vi "Bar Code Reader_v3.vi"() -> ()   [LabVIEW 2016]
uses:
  <vilib>/NXT/Block Support/NXT_OutputPort.ctl
  <vilib>/NXT/Block Support/NXT_InputPort.ctl
  <vilib>/NXT/Dual Mode Library/Sensors/EV3_Color_Color.vi
  <vilib>/NXT/NXTIO Xnodes/NXTIONodeSubVIs/NXTMoveMotors.vi
  <vilib>/NXT/NXTIO Xnodes/NXTIONodeSubVIs/NXTMotorRunDistance.vi
  <vilib>/NXT/Dual Mode Library/Waits/Wait_Num.vi
  <vilib>/NXT/Subs/LVHSConnector.ctl
  <vilib>/NXT/NXTIO Xnodes/AddressXNode/NXTIOAddress.xnode
  <vilib>/NXT/NXTIO Xnodes/NXTIOXNode/NXTIO.xnode
  <vilib>/NXT/LegoClasses/BrickReference/BrickReference.lvclass
panel:
  out "Error Message":string
  out "Total Marbles":dbl
  out "Small/HDPE 4":dbl
  out "Large/Steel 4":dbl
  out "Material 4":string
  out "Small/HDPE 3":dbl
  out "Large/Steel 3":dbl
  out "Material 3":string
  out "Small/HDPE 2":dbl
  out "Large/Steel 2":dbl
  out "Material 2":string
  out "Small/HDPE 1":dbl
  out "Large/Steel 1":dbl
  out "String 3":string
  out "String 2":string
  out "Material 1":string
  out "String":string
  out "Numeric":dbl
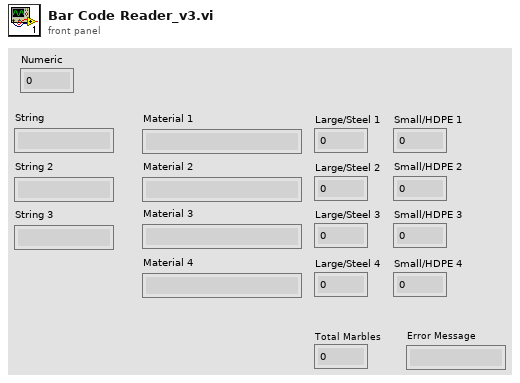
[diagram p1: front panel]
types:
  T1 = typedef "ColorSensorColors.ctl" = enum16{"No Color", "Black", "Blue", "Green", "Yellow", "Red", "White", "Brown"}
  T2 = typedef "NXT_OutputPort.ctl" = u8
  T3 = typedef "LVHSConnector.ctl" = refnum<class "BrickReference.lvclass">
  T4 = typedef "NXT_InputPort.ctl" = u32
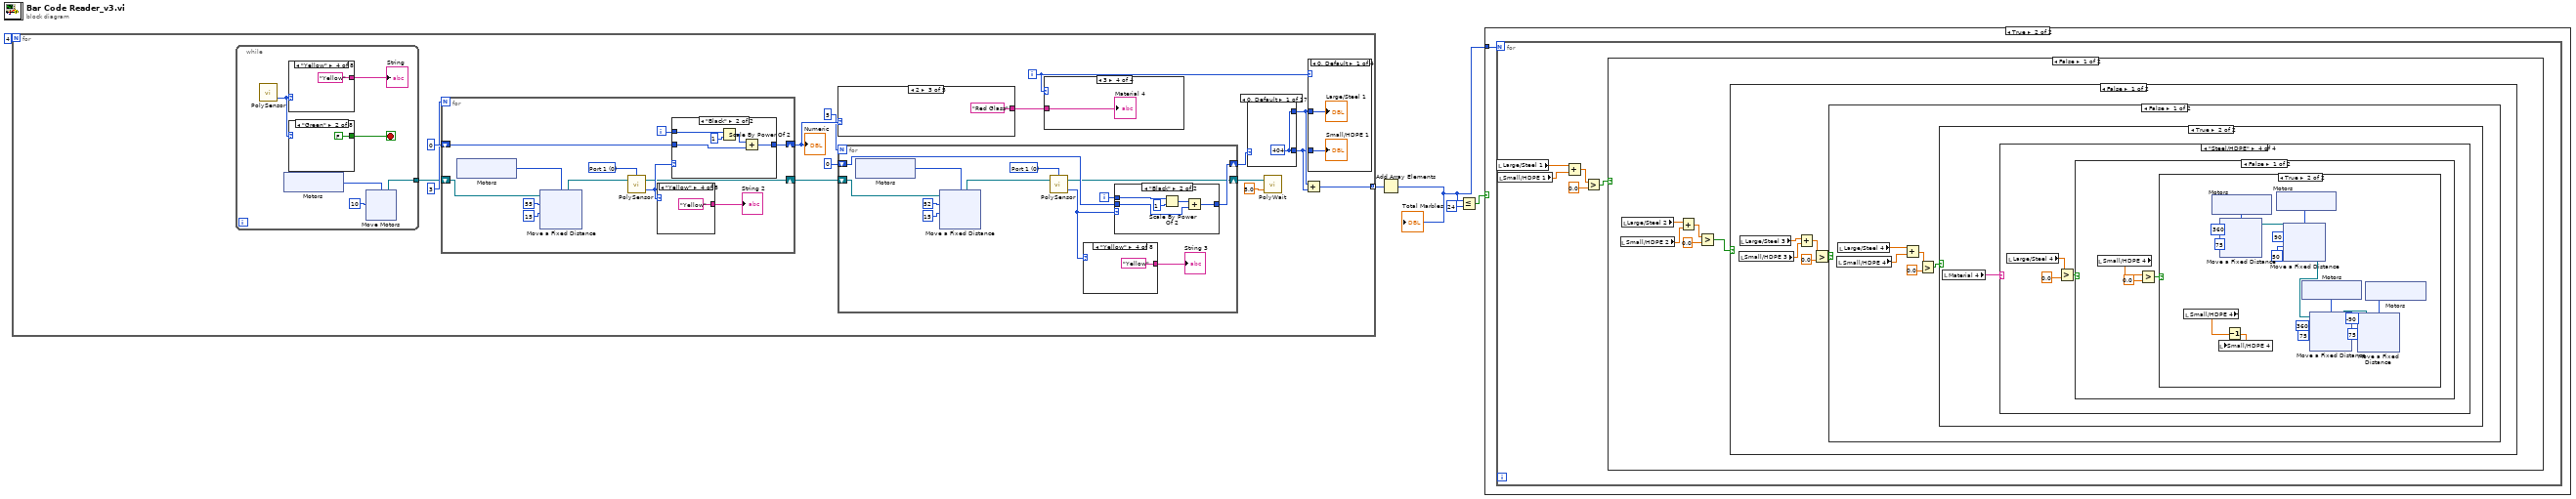
[diagram p0: block diagram]
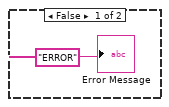
[diagram p2: hidden frame]
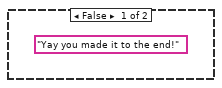
[diagram p3: hidden frame]
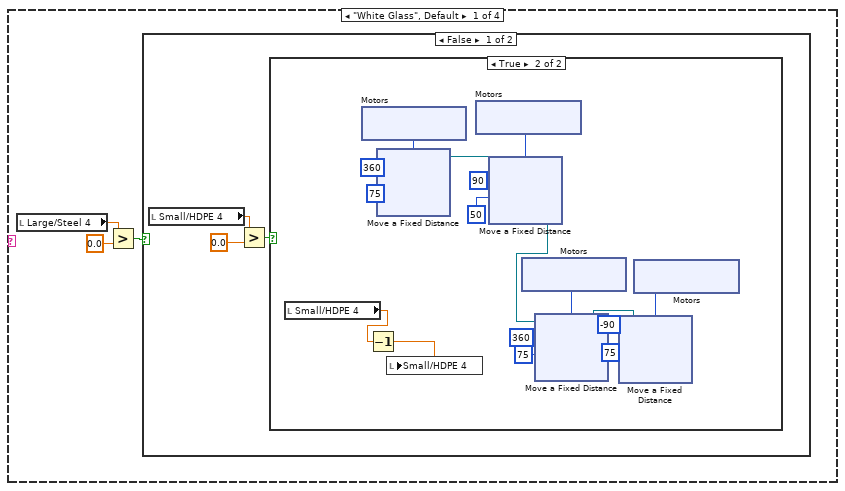
[diagram p4: hidden frame]
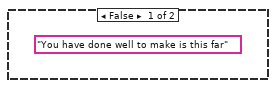
[diagram p5: hidden frame]
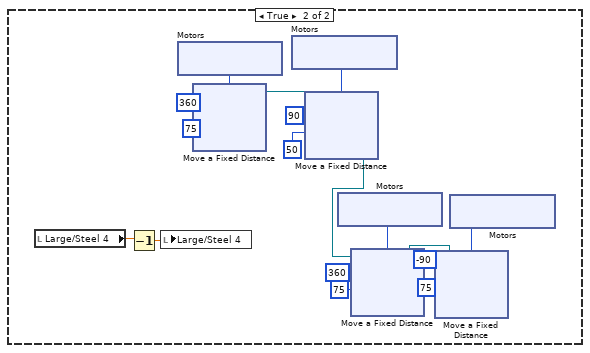
[diagram p6: hidden frame]
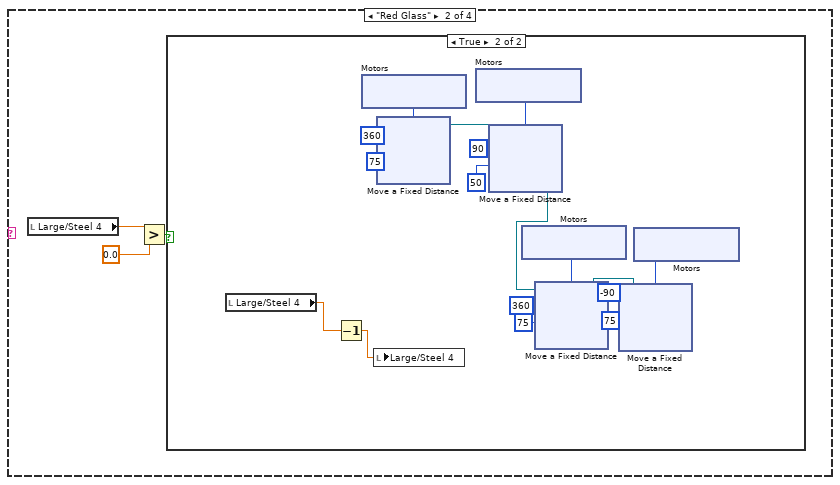
[diagram p7: hidden frame]
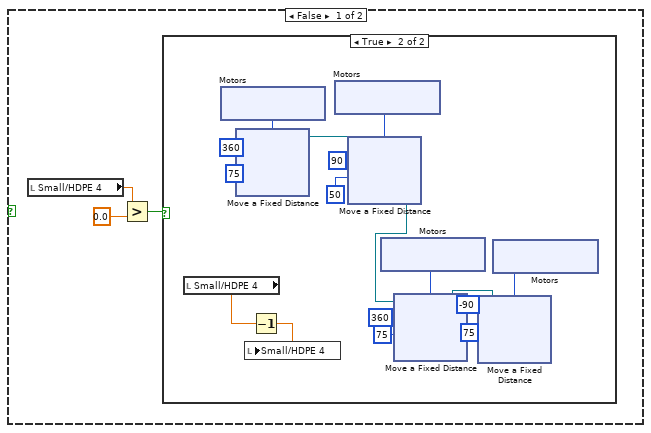
[diagram p8: hidden frame]
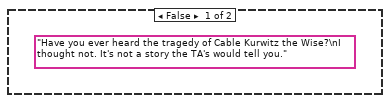
[diagram p9: hidden frame]
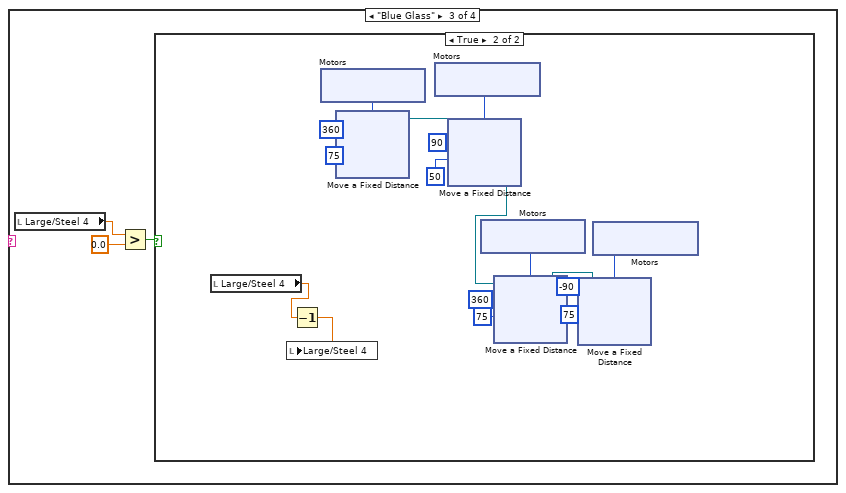
[diagram p10: hidden frame]
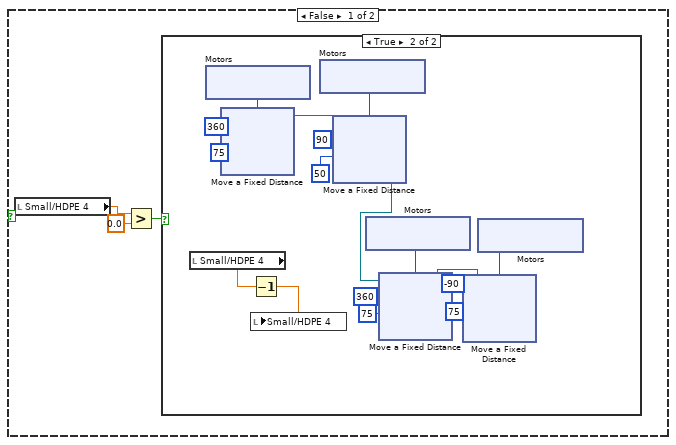
[diagram p11: hidden frame]
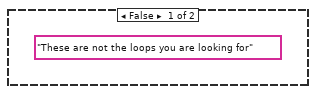
[diagram p12: hidden frame]
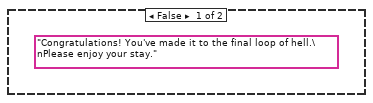
[diagram p13: hidden frame]
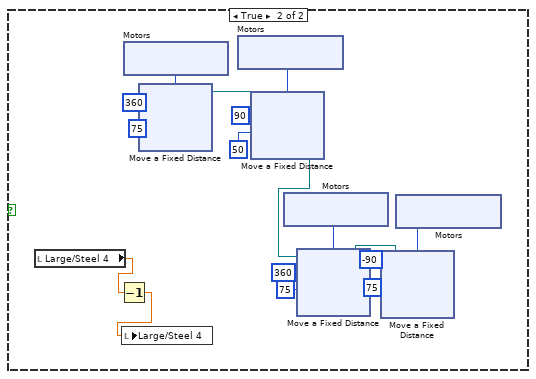
[diagram p14: hidden frame]
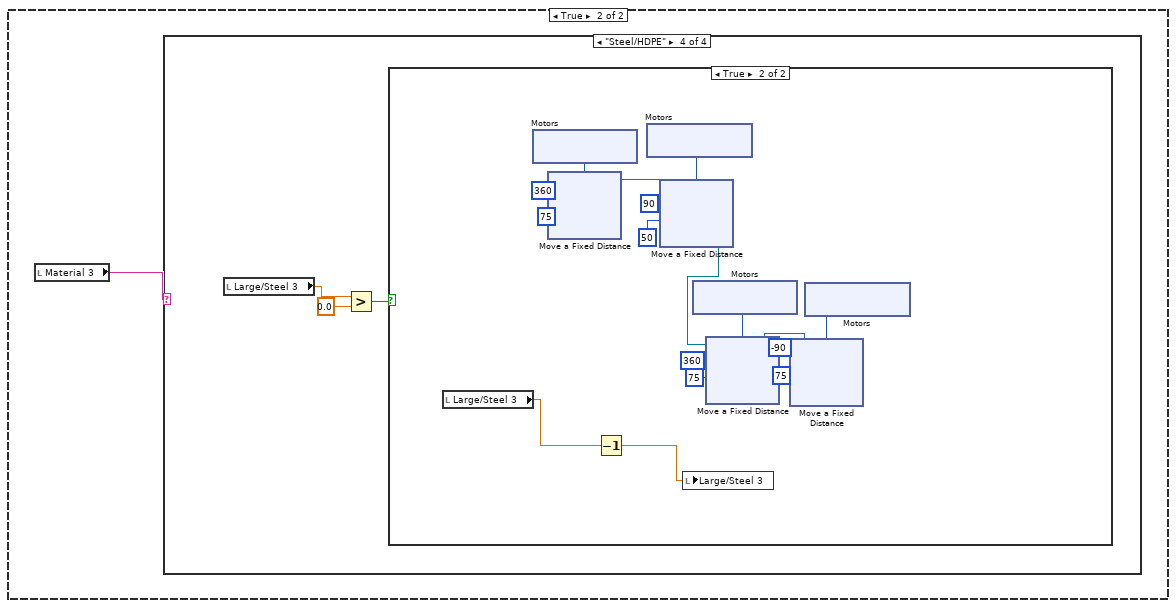
[diagram p15: hidden frame]
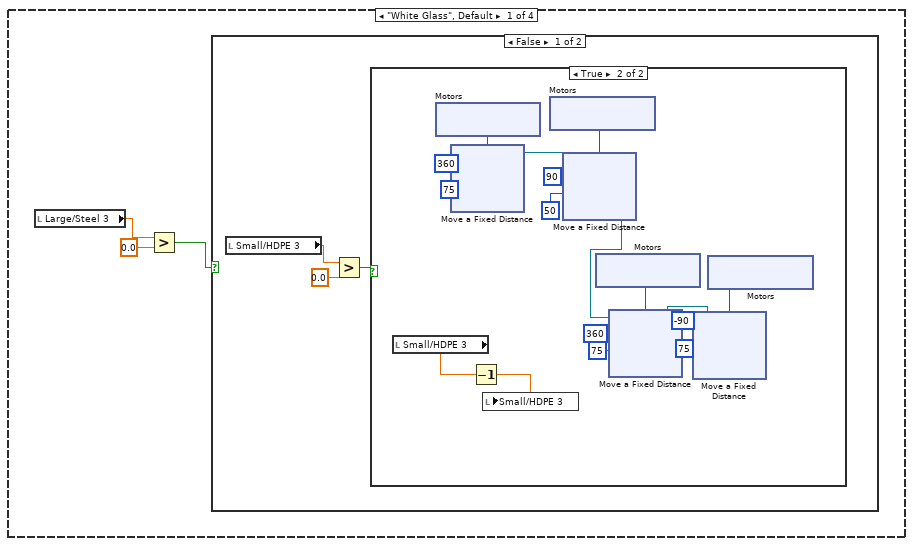
[diagram p16: hidden frame]
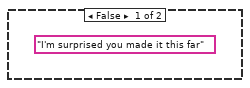
[diagram p17: hidden frame]
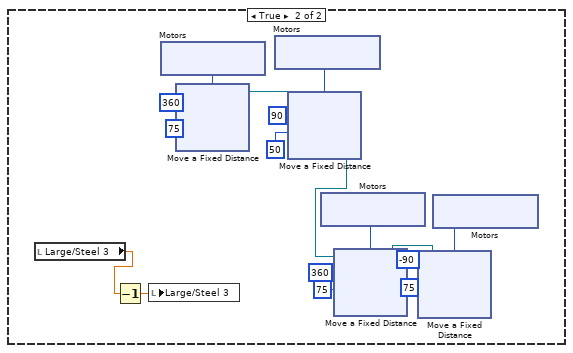
[diagram p18: hidden frame]
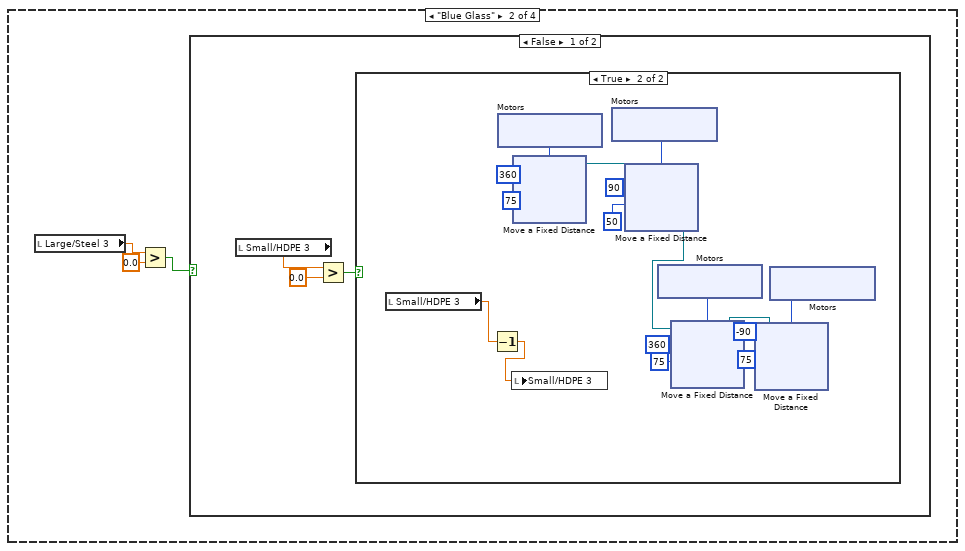
[diagram p19: hidden frame]
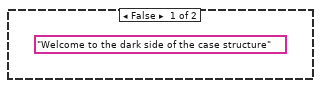
[diagram p20: hidden frame]
diagram:
  n1 = for {
    N: 4 -> [_]
    tunnel: [w6] -> w4 mode=indexing
    i -> [w11]
    n2 = while {
      tunnel: [w109] -> w18
      stop <- w113 stop-if-true
      n3 = call-poly <vilib>:"PolySensor.vi"() -> ("Detected Color"=w111:T1)  [unwired: 3 in, 1 out]
      n4 = xnode "Motors"() -> ("Motor"=w108:T2)
      n5 = case shown="\"Yellow\"" w111 {
        tunnel: ["No Color" "Blue" "Green" "Yellow" "Red" "White" "Brown" "Black"] -> w112
        frame "No Color", Default {
        }
        frame "Blue" {
        }
        frame "Green" {
        }
        frame "Yellow" {
        }
        frame "Red" {
        }
        frame "White" {
        }
        frame "Brown" {
        }
        frame "Black" {
        }
      }
      "String" <- w112
      n6 = case shown="\"Green\"" w111 {
        tunnel: [FALSE FALSE FALSE FALSE FALSE FALSE FALSE TRUE] -> w113
        frame "No Color", Default {
        }
        frame "Green" {
        }
        frame "Yellow" {
        }
        frame "Red" {
        }
        frame "White" {
        }
        frame "Brown" {
        }
        frame "Blue" {
        }
        frame "Black" {
        }
      }
      n7 = xnode "Move Motors"("Power/Speed 1"=i8 10, "Motors"=w108) -> ("NXT/EV3"=w109:T3)  [unwired: 1 in]
    }
    n8 = for {
      N: 3 -> [_]
      shift-right: [w149] -> w17
      shift-left: 0 -> [w148]
      shift-right: [w144] -> w13
      shift-left: w18 -> [w141]
      i -> [w145]
      w138 = T4 0 items=["Port 1", "Port 2", "Port 3", "Port 4"] ("Port (Port 1)")
      n9 = xnode "Motors"() -> ("Motor"=w139:T2)
      n10 = xnode "Move a Fixed Distance"("Speed 1"=i8 15, "Distance 1"=55, "Motors"=w139, "NXT/EV3"=w141) -> ("NXT/EV3"=w140:T3)
      n11 = call-poly <vilib>:"PolySensor.vi"("NXT/EV3"=w140, "Port (Port 1)"=w138) -> ("Detected Color"=w146:T1, "NXT/EV3"=w144:T3)  [unwired: 1 in]
      n12 = case shown="\"Yellow\"" w146 {
        tunnel: ["No Color" "Blue" "Green" "Yellow" "Red" "White" "Brown" "Black"] -> w147
        frame "No Color", Default {
        }
        frame "Blue" {
        }
        frame "Green" {
        }
        frame "Yellow" {
        }
        frame "Red" {
        }
        frame "White" {
        }
        frame "Brown" {
        }
        frame "Black" {
        }
      }
      "String 2" <- w147
      n13 = case shown="\"Black\"" w146 {
        tunnel: w145 -> [_ w173]
        tunnel: [w169 w171] -> w149
        tunnel: w148 -> [w169 w170]
        frame "White", Default {
        }
        frame "Black" {
          n14 = Scale By Power Of 2(n=w173, x=1) -> (x*2^n=w172:i32)
          n15 = Add(x=w172, y=w170) -> (x+y=w171:i32)
        }
      }
    }
    "Numeric" <- w17
    n16 = case shown="2" w17 {
      tunnel: ["Something has gone wrong" "White Glass" "Red Glass" "Blue Glass" "Steel/HDPE"] -> w16
      frame 0, Default {
      }
      frame 1 {
      }
      frame 2 {
      }
      frame 3 {
      }
      frame 4 {
      }
    }
    n17 = for {
      N: 5 -> [_]
      shift-right: [w77] -> w12
      shift-left: 0 -> [w76]
      shift-right: [w72] -> w10
      shift-left: w13 -> [w69]
      i -> [w73]
      w66 = T4 0 items=["Port 1", "Port 2", "Port 3", "Port 4"] ("Port (Port 1)")
      n18 = xnode "Motors"() -> ("Motor"=w67:T2)
      n19 = xnode "Move a Fixed Distance"("Speed 1"=i8 15, "Distance 1"=52, "Motors"=w67, "NXT/EV3"=w69) -> ("NXT/EV3"=w68:T3)
      n20 = call-poly <vilib>:"PolySensor.vi"("NXT/EV3"=w68, "Port (Port 1)"=w66) -> ("Detected Color"=w74:T1, "NXT/EV3"=w72:T3)  [unwired: 1 in]
      n21 = case shown="\"Yellow\"" w74 {
        tunnel: ["No Color" "Blue" "Green" "Yellow" "Red" "White" "Brown" "Black"] -> w75
        frame "No Color", Default {
        }
        frame "Blue" {
        }
        frame "Green" {
        }
        frame "Yellow" {
        }
        frame "Red" {
        }
        frame "White" {
        }
        frame "Brown" {
        }
        frame "Black" {
        }
      }
      "String 3" <- w75
      n22 = case shown="\"Black\"" w74 {
        tunnel: w73 -> [_ w101]
        tunnel: [w97 w99] -> w77
        tunnel: w76 -> [w97 w98]
        frame "White", Default {
        }
        frame "Black" {
          n23 = Scale By Power Of 2(n=w101, x=1) -> (x*2^n=w100:i32)
          n24 = Add(x=w100, y=w98) -> (x+y=w99:i32)
        }
      }
    }
    n25 = case shown="3" w11 {
      tunnel: w16 -> [w29 w30 w31 w32]
      frame 0, Default {
        "Material 1" <- w29
      }
      frame 1 {
        "Material 2" <- w30
      }
      frame 2 {
        "Material 3" <- w31
      }
      frame 3 {
        "Material 4" <- w32
      }
    }
    n26 = case shown="0, Default" w12 {
      tunnel: [w33 0 1 2 3 0 1 2 3 0 1 2 3 0 1 2 3] -> w8
      tunnel: [w33 0 0 0 0 1 1 1 1 2 2 2 2 3 3 3 3] -> w7
      frame 0, Default {
        w33 = 404
      }
      frame 1 {
      }
      frame 2 {
      }
      frame 3 {
      }
      frame 4 {
      }
      frame 5 {
      }
      frame 6 {
      }
      frame 7 {
      }
      frame 8 {
      }
      frame 9 {
      }
      frame 10 {
      }
      frame 11 {
      }
      frame 12 {
      }
      frame 13 {
      }
      frame 14 {
      }
      frame 15 {
      }
      frame 16 {
      }
    }
    n27 = call-poly <vilib>:"PolyWait.vi"("Time (1 sec)"=sgl 5.0, "NXT/EV3"=w10) -> ()  [unwired: 2 in, 1 out]
    n28 = Add(x=w8, y=w7) -> (x+y=w6:i32)
    n29 = case shown="0, Default" w11 {
      tunnel: w8 -> [w22 w23 w25 w27]
      tunnel: w7 -> [w21 w24 w26 w28]
      frame 0, Default {
        "Small/HDPE 1" <- w21
        "Large/Steel 1" <- w22
      }
      frame 1 {
        "Large/Steel 2" <- w23
        "Small/HDPE 2" <- w24
      }
      frame 2 {
        "Large/Steel 3" <- w25
        "Small/HDPE 3" <- w26
      }
      frame 3 {
        "Large/Steel 4" <- w27
        "Small/HDPE 4" <- w28
      }
    }
  }
  n30 = Add Array Elements(numeric array=w4) -> (sum=w3:i32)
  "Total Marbles" <- w3
  n31 = Less Or Equal?(x=w3, y=24) -> (x <= y?=w1:bool)
  n32 = case shown="True" w1 {
    tunnel: w3 -> [_ w176]
    frame False {
      "Error Message" <- "ERROR"
    }
    frame True {
      n33 = for {
        N: w176 -> [_]
        n34 = local read "Large/Steel 1"() -> (w181:dbl)
        n35 = local read "Small/HDPE 1"() -> (w180:dbl)
        n36 = Add(x=w181, y=w180) -> (x+y=w179:dbl)
        n37 = Greater?(x=w179, y=0.0) -> (0:w177:bool)
        n38 = case shown="False" w177 {
          frame False {
            n39 = local read "Small/HDPE 2"() -> (w184:dbl)
            n40 = local read "Large/Steel 2"() -> (w183:dbl)
            n41 = Add(x=w183, y=w184) -> (x+y=w186:dbl)
            n42 = Greater?(x=w186, y=0.0) -> (0:w182:bool)
            n43 = case shown="False" w182 {
              frame False {
                n44 = local read "Small/HDPE 3"() -> (w188:dbl)
                n45 = local read "Large/Steel 3"() -> (w189:dbl)
                n46 = Add(x=w189, y=w188) -> (x+y=w191:dbl)
                n47 = Greater?(x=w191, y=0.0) -> (0:w187:bool)
                n48 = case shown="False" w187 {
                  frame False {
                    n49 = local read "Small/HDPE 4"() -> (w193:dbl)
                    n50 = local read "Large/Steel 4"() -> (w194:dbl)
                    n51 = Add(x=w194, y=w193) -> (x+y=w196:dbl)
                    n52 = Greater?(x=w196, y=0.0) -> (0:w192:bool)
                    n53 = case shown="True" w192 {
                      frame False {
                        (unwired) "Yay you made it to the end!"
                      }
                      frame True {
                        n54 = local read "Material 4"() -> (w197:string)
                        n55 = case shown="\"Steel/HDPE\"" w197 {
                          frame "White Glass", Default {
                            n56 = local read "Large/Steel 4"() -> (w199:dbl)
                            n57 = Greater?(x=w199, y=0.0) -> (0:w200:bool)
                            n58 = case shown="False" w200 {
                              frame False {
                                n59 = local read "Small/HDPE 4"() -> (w202:dbl)
                                n60 = Greater?(x=w202, y=0.0) -> (0:w203:bool)
                                n61 = case shown="True" w203 {
                                frame False {
                                (unwired) "You have done well to make is this far"
                                }
                                frame True {
                                n62 = local read "Small/HDPE 4"() -> (w205:dbl)
                                n63 = xnode "Motors"() -> ("Motor"=w206:T2)
                                n64 = Decrement(x=w205) -> (x-1=w204:dbl)
                                n65 = xnode "Move a Fixed Distance"("Speed 1"=i8 75, "Distance 1"=360, "Motors"=w206) -> ("NXT/EV3"=w209:T3)  [unwired: 1 in]
                                n66 = local write "Small/HDPE 4"(w204) -> ()
                                n67 = xnode "Motors"() -> ("Motor"=w210:T2)
                                n68 = xnode "Move a Fixed Distance"("Speed 1"=i8 50, "Distance 1"=90, "Motors"=w210, "NXT/EV3"=w209) -> ("NXT/EV3"=w220:T3)
                                n69 = xnode "Motors"() -> ("Motor"=w216:T2)
                                n70 = xnode "Move a Fixed Distance"("Speed 1"=i8 75, "Distance 1"=360, "Motors"=w216, "NXT/EV3"=w220) -> ("NXT/EV3"=w219:T3)
                                n71 = xnode "Motors"() -> ("Motor"=w213:T2)
                                n72 = xnode "Move a Fixed Distance"("Speed 1"=i8 75, "Distance 1"=-90, "Motors"=w213, "NXT/EV3"=w219) -> ()  [unwired: 1 out]
                                }
                                }
                              }
                              frame True {
                                n73 = local read "Large/Steel 4"() -> (w266:dbl)
                                n74 = Decrement(x=w266) -> (x-1=w265:dbl)
                                n75 = local write "Large/Steel 4"(w265) -> ()
                                n76 = xnode "Motors"() -> ("Motor"=w267:T2)
                                n77 = xnode "Move a Fixed Distance"("Speed 1"=i8 75, "Distance 1"=360, "Motors"=w267) -> ("NXT/EV3"=w270:T3)  [unwired: 1 in]
                                n78 = xnode "Motors"() -> ("Motor"=w271:T2)
                                n79 = xnode "Move a Fixed Distance"("Speed 1"=i8 50, "Distance 1"=90, "Motors"=w271, "NXT/EV3"=w270) -> ("NXT/EV3"=w281:T3)
                                n80 = xnode "Motors"() -> ("Motor"=w277:T2)
                                n81 = xnode "Move a Fixed Distance"("Speed 1"=i8 75, "Distance 1"=360, "Motors"=w277, "NXT/EV3"=w281) -> ("NXT/EV3"=w280:T3)
                                n82 = xnode "Motors"() -> ("Motor"=w274:T2)
                                n83 = xnode "Move a Fixed Distance"("Speed 1"=i8 75, "Distance 1"=-90, "Motors"=w274, "NXT/EV3"=w280) -> ()  [unwired: 1 out]
                              }
                            }
                          }
                          frame "Red Glass" {
                            n84 = local read "Large/Steel 4"() -> (w327:dbl)
                            n85 = Greater?(x=w327, y=0.0) -> (0:w328:bool)
                            n86 = case shown="True" w328 {
                              frame False {
                                n87 = local read "Small/HDPE 4"() -> (w329:dbl)
                                n88 = Greater?(x=w329, y=0.0) -> (0:w331:bool)
                                n89 = case shown="True" w331 {
                                frame False {
                                (unwired) "Have you ever heard the tragedy of Cable Kurwitz the Wise?\nI thought not. It's not a story the TA's would tell you."
                                }
                                frame True {
                                n90 = local read "Small/HDPE 4"() -> (w333:dbl)
                                n91 = xnode "Motors"() -> ("Motor"=w348:T2)
                                n92 = xnode "Move a Fixed Distance"("Speed 1"=i8 75, "Distance 1"=360, "Motors"=w348) -> ("NXT/EV3"=w345:T3)  [unwired: 1 in]
                                n93 = Decrement(x=w333) -> (x-1=w332:dbl)
                                n94 = local write "Small/HDPE 4"(w332) -> ()
                                n95 = xnode "Motors"() -> ("Motor"=w344:T2)
                                n96 = xnode "Move a Fixed Distance"("Speed 1"=i8 50, "Distance 1"=90, "Motors"=w344, "NXT/EV3"=w345) -> ("NXT/EV3"=w334:T3)
                                n97 = xnode "Motors"() -> ("Motor"=w338:T2)
                                n98 = xnode "Move a Fixed Distance"("Speed 1"=i8 75, "Distance 1"=360, "Motors"=w338, "NXT/EV3"=w334) -> ("NXT/EV3"=w335:T3)
                                n99 = xnode "Motors"() -> ("Motor"=w341:T2)
                                n100 = xnode "Move a Fixed Distance"("Speed 1"=i8 75, "Distance 1"=-90, "Motors"=w341, "NXT/EV3"=w335) -> ()  [unwired: 1 out]
                                }
                                }
                              }
                              frame True {
                                n101 = local read "Large/Steel 4"() -> (w394:dbl)
                                n102 = Decrement(x=w394) -> (x-1=w393:dbl)
                                n103 = xnode "Motors"() -> ("Motor"=w395:T2)
                                n104 = local write "Large/Steel 4"(w393) -> ()
                                n105 = xnode "Move a Fixed Distance"("Speed 1"=i8 75, "Distance 1"=360, "Motors"=w395) -> ("NXT/EV3"=w398:T3)  [unwired: 1 in]
                                n106 = xnode "Motors"() -> ("Motor"=w399:T2)
                                n107 = xnode "Move a Fixed Distance"("Speed 1"=i8 50, "Distance 1"=90, "Motors"=w399, "NXT/EV3"=w398) -> ("NXT/EV3"=w409:T3)
                                n108 = xnode "Motors"() -> ("Motor"=w405:T2)
                                n109 = xnode "Move a Fixed Distance"("Speed 1"=i8 75, "Distance 1"=360, "Motors"=w405, "NXT/EV3"=w409) -> ("NXT/EV3"=w408:T3)
                                n110 = xnode "Motors"() -> ("Motor"=w402:T2)
                                n111 = xnode "Move a Fixed Distance"("Speed 1"=i8 75, "Distance 1"=-90, "Motors"=w402, "NXT/EV3"=w408) -> ()  [unwired: 1 out]
                              }
                            }
                          }
                          frame "Blue Glass" {
                            n112 = local read "Large/Steel 4"() -> (w456:dbl)
                            n113 = Greater?(x=w456, y=0.0) -> (0:w455:bool)
                            n114 = case shown="True" w455 {
                              frame False {
                                n115 = local read "Small/HDPE 4"() -> (w458:dbl)
                                n116 = Greater?(x=w458, y=0.0) -> (0:w459:bool)
                                n117 = case shown="True" w459 {
                                frame False {
                                (unwired) "These are not the loops you are looking for"
                                }
                                frame True {
                                n118 = local read "Small/HDPE 4"() -> (w461:dbl)
                                n119 = xnode "Motors"() -> ("Motor"=w462:T2)
                                n120 = xnode "Move a Fixed Distance"("Speed 1"=i8 75, "Distance 1"=360, "Motors"=w462) -> ("NXT/EV3"=w465:T3)  [unwired: 1 in]
                                n121 = Decrement(x=w461) -> (x-1=w460:dbl)
                                n122 = local write "Small/HDPE 4"(w460) -> ()
                                n123 = xnode "Motors"() -> ("Motor"=w466:T2)
                                n124 = xnode "Move a Fixed Distance"("Speed 1"=i8 50, "Distance 1"=90, "Motors"=w466, "NXT/EV3"=w465) -> ("NXT/EV3"=w476:T3)
                                n125 = xnode "Motors"() -> ("Motor"=w472:T2)
                                n126 = xnode "Move a Fixed Distance"("Speed 1"=i8 75, "Distance 1"=360, "Motors"=w472, "NXT/EV3"=w476) -> ("NXT/EV3"=w475:T3)
                                n127 = xnode "Motors"() -> ("Motor"=w469:T2)
                                n128 = xnode "Move a Fixed Distance"("Speed 1"=i8 75, "Distance 1"=-90, "Motors"=w469, "NXT/EV3"=w475) -> ()  [unwired: 1 out]
                                }
                                }
                              }
                              frame True {
                                n129 = local read "Large/Steel 4"() -> (w522:dbl)
                                n130 = Decrement(x=w522) -> (x-1=w521:dbl)
                                n131 = local write "Large/Steel 4"(w521) -> ()
                                n132 = xnode "Motors"() -> ("Motor"=w523:T2)
                                n133 = xnode "Move a Fixed Distance"("Speed 1"=i8 75, "Distance 1"=360, "Motors"=w523) -> ("NXT/EV3"=w526:T3)  [unwired: 1 in]
                                n134 = xnode "Motors"() -> ("Motor"=w527:T2)
                                n135 = xnode "Move a Fixed Distance"("Speed 1"=i8 50, "Distance 1"=90, "Motors"=w527, "NXT/EV3"=w526) -> ("NXT/EV3"=w537:T3)
                                n136 = xnode "Motors"() -> ("Motor"=w533:T2)
                                n137 = xnode "Move a Fixed Distance"("Speed 1"=i8 75, "Distance 1"=360, "Motors"=w533, "NXT/EV3"=w537) -> ("NXT/EV3"=w536:T3)
                                n138 = xnode "Motors"() -> ("Motor"=w530:T2)
                                n139 = xnode "Move a Fixed Distance"("Speed 1"=i8 75, "Distance 1"=-90, "Motors"=w530, "NXT/EV3"=w536) -> ()  [unwired: 1 out]
                              }
                            }
                          }
                          frame "Steel/HDPE" {
                            n140 = local read "Large/Steel 4"() -> (w583:dbl)
                            n141 = Greater?(x=w583, y=0.0) -> (0:w584:bool)
                            n142 = case shown="False" w584 {
                              frame False {
                                n143 = local read "Small/HDPE 4"() -> (w586:dbl)
                                n144 = Greater?(x=w586, y=0.0) -> (0:w587:bool)
                                n145 = case shown="True" w587 {
                                frame False {
                                (unwired) "Congratulations! You've made it to the final loop of hell.\nPlease enjoy your stay."
                                }
                                frame True {
                                n146 = local read "Small/HDPE 4"() -> (w589:dbl)
                                n147 = xnode "Motors"() -> ("Motor"=w590:T2)
                                n148 = xnode "Move a Fixed Distance"("Speed 1"=i8 75, "Distance 1"=360, "Motors"=w590) -> ("NXT/EV3"=w593:T3)  [unwired: 1 in]
                                n149 = Decrement(x=w589) -> (x-1=w588:dbl)
                                n150 = local write "Small/HDPE 4"(w588) -> ()
                                n151 = xnode "Motors"() -> ("Motor"=w594:T2)
                                n152 = xnode "Move a Fixed Distance"("Speed 1"=i8 50, "Distance 1"=90, "Motors"=w594, "NXT/EV3"=w593) -> ("NXT/EV3"=w604:T3)
                                n153 = xnode "Motors"() -> ("Motor"=w600:T2)
                                n154 = xnode "Move a Fixed Distance"("Speed 1"=i8 75, "Distance 1"=360, "Motors"=w600, "NXT/EV3"=w604) -> ("NXT/EV3"=w603:T3)
                                n155 = xnode "Motors"() -> ("Motor"=w597:T2)
                                n156 = xnode "Move a Fixed Distance"("Speed 1"=i8 75, "Distance 1"=-90, "Motors"=w597, "NXT/EV3"=w603) -> ()  [unwired: 1 out]
                                }
                                }
                              }
                              frame True {
                                n157 = local read "Large/Steel 4"() -> (w650:dbl)
                                n158 = Decrement(x=w650) -> (x-1=w649:dbl)
                                n159 = local write "Large/Steel 4"(w649) -> ()
                                n160 = xnode "Motors"() -> ("Motor"=w651:T2)
                                n161 = xnode "Move a Fixed Distance"("Speed 1"=i8 75, "Distance 1"=360, "Motors"=w651) -> ("NXT/EV3"=w654:T3)  [unwired: 1 in]
                                n162 = xnode "Motors"() -> ("Motor"=w655:T2)
                                n163 = xnode "Move a Fixed Distance"("Speed 1"=i8 50, "Distance 1"=90, "Motors"=w655, "NXT/EV3"=w654) -> ("NXT/EV3"=w665:T3)
                                n164 = xnode "Motors"() -> ("Motor"=w661:T2)
                                n165 = xnode "Move a Fixed Distance"("Speed 1"=i8 75, "Distance 1"=360, "Motors"=w661, "NXT/EV3"=w665) -> ("NXT/EV3"=w664:T3)
                                n166 = xnode "Motors"() -> ("Motor"=w658:T2)
                                n167 = xnode "Move a Fixed Distance"("Speed 1"=i8 75, "Distance 1"=-90, "Motors"=w658, "NXT/EV3"=w664) -> ()  [unwired: 1 out]
                              }
                            }
                          }
                        }
                      }
                    }
                  }
                  frame True {
                    n168 = local read "Material 3"() -> (w710:string)
                    n169 = case shown="\"Steel/HDPE\"" w710 {
                      frame "White Glass", Default {
                        n170 = local read "Large/Steel 3"() -> (w713:dbl)
                        n171 = Greater?(x=w713, y=0.0) -> (0:w711:bool)
                        n172 = case shown="False" w711 {
                          frame False {
                            n173 = local read "Small/HDPE 3"() -> (w715:dbl)
                            n174 = Greater?(x=w715, y=0.0) -> (0:w716:bool)
                            n175 = case shown="True" w716 {
                              frame False {
                                (unwired) "I'm surprised you made it this far"
                              }
                              frame True {
                                n176 = local read "Small/HDPE 3"() -> (w718:dbl)
                                n177 = xnode "Motors"() -> ("Motor"=w719:T2)
                                n178 = xnode "Move a Fixed Distance"("Speed 1"=i8 75, "Distance 1"=360, "Motors"=w719) -> ("NXT/EV3"=w722:T3)  [unwired: 1 in]
                                n179 = Decrement(x=w718) -> (x-1=w717:dbl)
                                n180 = local write "Small/HDPE 3"(w717) -> ()
                                n181 = xnode "Motors"() -> ("Motor"=w723:T2)
                                n182 = xnode "Move a Fixed Distance"("Speed 1"=i8 50, "Distance 1"=90, "Motors"=w723, "NXT/EV3"=w722) -> ("NXT/EV3"=w733:T3)
                                n183 = xnode "Motors"() -> ("Motor"=w729:T2)
                                n184 = xnode "Move a Fixed Distance"("Speed 1"=i8 75, "Distance 1"=360, "Motors"=w729, "NXT/EV3"=w733) -> ("NXT/EV3"=w732:T3)
                                n185 = xnode "Motors"() -> ("Motor"=w726:T2)
                                n186 = xnode "Move a Fixed Distance"("Speed 1"=i8 75, "Distance 1"=-90, "Motors"=w726, "NXT/EV3"=w732) -> ()  [unwired: 1 out]
                              }
                            }
                          }
                          frame True {
                            n187 = local read "Large/Steel 3"() -> (w779:dbl)
                            n188 = Decrement(x=w779) -> (x-1=w778:dbl)
                            n189 = local write "Large/Steel 3"(w778) -> ()
                            n190 = xnode "Motors"() -> ("Motor"=w780:T2)
                            n191 = xnode "Move a Fixed Distance"("Speed 1"=i8 75, "Distance 1"=360, "Motors"=w780) -> ("NXT/EV3"=w783:T3)  [unwired: 1 in]
                            n192 = xnode "Motors"() -> ("Motor"=w784:T2)
                            n193 = xnode "Move a Fixed Distance"("Speed 1"=i8 50, "Distance 1"=90, "Motors"=w784, "NXT/EV3"=w783) -> ("NXT/EV3"=w794:T3)
                            n194 = xnode "Motors"() -> ("Motor"=w790:T2)
                            n195 = xnode "Move a Fixed Distance"("Speed 1"=i8 75, "Distance 1"=360, "Motors"=w790, "NXT/EV3"=w794) -> ("NXT/EV3"=w793:T3)
                            n196 = xnode "Motors"() -> ("Motor"=w787:T2)
                            n197 = xnode "Move a Fixed Distance"("Speed 1"=i8 75, "Distance 1"=-90, "Motors"=w787, "NXT/EV3"=w793) -> ()  [unwired: 1 out]
                          }
                        }
                      }
                      frame "Blue Glass" {
                        n198 = local read "Large/Steel 3"() -> (w841:dbl)
                        n199 = Greater?(x=w841, y=0.0) -> (0:w839:bool)
                        n200 = case shown="False" w839 {
                          frame False {
                            n201 = local read "Small/HDPE 3"() -> (w844:dbl)
                            n202 = Greater?(x=w844, y=0.0) -> (0:w842:bool)
                            n203 = case shown="True" w842 {
                              frame False {
                                (unwired) "Welcome to the dark side of the case structure"
                              }
                              frame True {
                                n204 = local read "Small/HDPE 3"() -> (w846:dbl)
                                n205 = Decrement(x=w846) -> (x-1=w845:dbl)
                                n206 = xnode "Motors"() -> ("Motor"=w847:T2)
                                n207 = local write "Small/HDPE 3"(w845) -> ()
                                n208 = xnode "Move a Fixed Distance"("Speed 1"=i8 75, "Distance 1"=360, "Motors"=w847) -> ("NXT/EV3"=w850:T3)  [unwired: 1 in]
                                n209 = xnode "Motors"() -> ("Motor"=w851:T2)
                                n210 = xnode "Move a Fixed Distance"("Speed 1"=i8 50, "Distance 1"=90, "Motors"=w851, "NXT/EV3"=w850) -> ("NXT/EV3"=w861:T3)
                                n211 = xnode "Motors"() -> ("Motor"=w857:T2)
                                n212 = xnode "Move a Fixed Distance"("Speed 1"=i8 75, "Distance 1"=360, "Motors"=w857, "NXT/EV3"=w861) -> ("NXT/EV3"=w860:T3)
                                n213 = xnode "Motors"() -> ("Motor"=w854:T2)
                                n214 = xnode "Move a Fixed Distance"("Speed 1"=i8 75, "Distance 1"=-90, "Motors"=w854, "NXT/EV3"=w860) -> ()  [unwired: 1 out]
                              }
                            }
                          }
                          frame True {
                            n215 = local read "Large/Steel 3"() -> (w907:dbl)
                            n216 = xnode "Motors"() -> ("Motor"=w908:T2)
                            n217 = xnode "Move a Fixed Distance"("Speed 1"=i8 75, "Distance 1"=360, "Motors"=w908) -> ("NXT/EV3"=w911:T3)  [unwired: 1 in]
                            n218 = Decrement(x=w907) -> (x-1=w906:dbl)
                            n219 = local write "Large/Steel 3"(w906) -> ()
                            n220 = xnode "Motors"() -> ("Motor"=w912:T2)
                            n221 = xnode "Move a Fixed Distance"("Speed 1"=i8 50, "Distance 1"=90, "Motors"=w912, "NXT/EV3"=w911) -> ("NXT/EV3"=w922:T3)
                            n222 = xnode "Motors"() -> ("Motor"=w918:T2)
                            n223 = xnode "Move a Fixed Distance"("Speed 1"=i8 75, "Distance 1"=360, "Motors"=w918, "NXT/EV3"=w922) -> ("NXT/EV3"=w921:T3)
                            n224 = xnode "Motors"() -> ("Motor"=w915:T2)
                            n225 = xnode "Move a Fixed Distance"("Speed 1"=i8 75, "Distance 1"=-90, "Motors"=w915, "NXT/EV3"=w921) -> ()  [unwired: 1 out]
                          }
                        }
                      }
                      frame "Red Glass" {
                        n226 = local read "Large/Steel 3"() -> (w968:dbl)
                        n227 = Greater?(x=w968, y=0.0) -> (0:w969:bool)
                        n228 = case shown="True" w969 {
                          frame False {
                            n229 = local read "Small/HDPE 3"() -> (w971:dbl)
                            n230 = Greater?(x=w971, y=0.0) -> (0:w972:bool)
                            n231 = case shown="True" w972 {
                              frame False {
                                (unwired) "Two to the one to the one to the three"
                              }
                              frame True {
                                n232 = local read "Small/HDPE 3"() -> (w974:dbl)
                                n233 = Decrement(x=w974) -> (x-1=w973:dbl)
                                n234 = local write "Small/HDPE 3"(w973) -> ()
                                n235 = xnode "Motors"() -> ("Motor"=w975:T2)
                                n236 = xnode "Move a Fixed Distance"("Speed 1"=i8 75, "Distance 1"=360, "Motors"=w975) -> ("NXT/EV3"=w978:T3)  [unwired: 1 in]
                                n237 = xnode "Motors"() -> ("Motor"=w979:T2)
                                n238 = xnode "Move a Fixed Distance"("Speed 1"=i8 50, "Distance 1"=90, "Motors"=w979, "NXT/EV3"=w978) -> ("NXT/EV3"=w989:T3)
                                n239 = xnode "Motors"() -> ("Motor"=w985:T2)
                                n240 = xnode "Move a Fixed Distance"("Speed 1"=i8 75, "Distance 1"=360, "Motors"=w985, "NXT/EV3"=w989) -> ("NXT/EV3"=w988:T3)
                                n241 = xnode "Motors"() -> ("Motor"=w982:T2)
                                n242 = xnode "Move a Fixed Distance"("Speed 1"=i8 75, "Distance 1"=-90, "Motors"=w982, "NXT/EV3"=w988) -> ()  [unwired: 1 out]
                              }
                            }
                          }
                          frame True {
                            n243 = local read "Large/Steel 3"() -> (w1035:dbl)
                            n244 = Decrement(x=w1035) -> (x-1=w1034:dbl)
                            n245 = local write "Large/Steel 3"(w1034) -> ()
                            n246 = xnode "Motors"() -> ("Motor"=w1036:T2)
                            n247 = xnode "Move a Fixed Distance"("Speed 1"=i8 75, "Distance 1"=360, "Motors"=w1036) -> ("NXT/EV3"=w1039:T3)  [unwired: 1 in]
                            n248 = xnode "Motors"() -> ("Motor"=w1040:T2)
                            n249 = xnode "Move a Fixed Distance"("Speed 1"=i8 50, "Distance 1"=90, "Motors"=w1040, "NXT/EV3"=w1039) -> ("NXT/EV3"=w1050:T3)
                            n250 = xnode "Motors"() -> ("Motor"=w1046:T2)
                            n251 = xnode "Move a Fixed Distance"("Speed 1"=i8 75, "Distance 1"=360, "Motors"=w1046, "NXT/EV3"=w1050) -> ("NXT/EV3"=w1049:T3)
                            n252 = xnode "Motors"() -> ("Motor"=w1043:T2)
                            n253 = xnode "Move a Fixed Distance"("Speed 1"=i8 75, "Distance 1"=-90, "Motors"=w1043, "NXT/EV3"=w1049) -> ()  [unwired: 1 out]
                          }
                        }
                      }
                      frame "Steel/HDPE" {
                        n254 = local read "Large/Steel 3"() -> (w1096:dbl)
                        n255 = Greater?(x=w1096, y=0.0) -> (0:w1097:bool)
                        n256 = case shown="True" w1097 {
                          frame False {
                            n257 = local read "Small/HDPE 3"() -> (w1099:dbl)
                            n258 = Greater?(x=w1099, y=0.0) -> (0:w1100:bool)
                            n259 = case shown="True" w1100 {
                              frame False {
                                (unwired) "labview wouldnt let me copy the variables successfully\nso I had to write every single case structure by hand."
                              }
                              frame True {
                                n260 = local read "Small/HDPE 3"() -> (w1102:dbl)
                                n261 = xnode "Motors"() -> ("Motor"=w1117:T2)
                                n262 = Decrement(x=w1102) -> (x-1=w1101:dbl)
                                n263 = xnode "Move a Fixed Distance"("Speed 1"=i8 75, "Distance 1"=360, "Motors"=w1117) -> ("NXT/EV3"=w1114:T3)  [unwired: 1 in]
                                n264 = local write "Small/HDPE 3"(w1101) -> ()
                                n265 = xnode "Motors"() -> ("Motor"=w1113:T2)
                                n266 = xnode "Move a Fixed Distance"("Speed 1"=i8 50, "Distance 1"=90, "Motors"=w1113, "NXT/EV3"=w1114) -> ("NXT/EV3"=w1103:T3)
                                n267 = xnode "Motors"() -> ("Motor"=w1107:T2)
                                n268 = xnode "Move a Fixed Distance"("Speed 1"=i8 75, "Distance 1"=360, "Motors"=w1107, "NXT/EV3"=w1103) -> ("NXT/EV3"=w1104:T3)
                                n269 = xnode "Motors"() -> ("Motor"=w1110:T2)
                                n270 = xnode "Move a Fixed Distance"("Speed 1"=i8 75, "Distance 1"=-90, "Motors"=w1110, "NXT/EV3"=w1104) -> ()  [unwired: 1 out]
                              }
                            }
                          }
                          frame True {
                            n271 = local read "Large/Steel 3"() -> (w1163:dbl)
                            n272 = xnode "Motors"() -> ("Motor"=w1164:T2)
                            n273 = xnode "Move a Fixed Distance"("Speed 1"=i8 75, "Distance 1"=360, "Motors"=w1164) -> ("NXT/EV3"=w1167:T3)  [unwired: 1 in]
                            n274 = Decrement(x=w1163) -> (x-1=w1162:dbl)
                            n275 = xnode "Motors"() -> ("Motor"=w1168:T2)
                            n276 = xnode "Move a Fixed Distance"("Speed 1"=i8 50, "Distance 1"=90, "Motors"=w1168, "NXT/EV3"=w1167) -> ("NXT/EV3"=w1178:T3)
                            n277 = local write "Large/Steel 3"(w1162) -> ()
                            n278 = xnode "Motors"() -> ("Motor"=w1174:T2)
                            n279 = xnode "Move a Fixed Distance"("Speed 1"=i8 75, "Distance 1"=360, "Motors"=w1174, "NXT/EV3"=w1178) -> ("NXT/EV3"=w1177:T3)
                            n280 = xnode "Motors"() -> ("Motor"=w1171:T2)
                            n281 = xnode "Move a Fixed Distance"("Speed 1"=i8 75, "Distance 1"=-90, "Motors"=w1171, "NXT/EV3"=w1177) -> ()  [unwired: 1 out]
                          }
                        }
                      }
                    }
                  }
                }
              }
              frame True {
                n282 = local read "Material 2"() -> (w1223:string)
                n283 = case shown="\"Steel/HDPE\"" w1223 {
                  frame "White Glass", Default {
                    n284 = local read "Large/Steel 2"() -> (w1226:dbl)
                    n285 = Greater?(x=w1226, y=0.0) -> (0:w1224:bool)
                    n286 = case shown="True" w1224 {
                      frame False {
                        n287 = local read "Small/HDPE 2"() -> (w1229:dbl)
                        n288 = Greater?(x=w1229, y=0.0) -> (0:w1227:bool)
                        n289 = case shown="True" w1227 {
                          frame False {
                            (unwired) "howdy random TA"
                          }
                          frame True {
                            n290 = local read "Small/HDPE 2"() -> (w1231:dbl)
                            n291 = Decrement(x=w1231) -> (x-1=w1230:dbl)
                            n292 = xnode "Motors"() -> ("Motor"=w1246:T2)
                            n293 = xnode "Move a Fixed Distance"("Speed 1"=i8 75, "Distance 1"=360, "Motors"=w1246) -> ("NXT/EV3"=w1243:T3)  [unwired: 1 in]
                            n294 = local write "Small/HDPE 2"(w1230) -> ()
                            n295 = xnode "Motors"() -> ("Motor"=w1242:T2)
                            n296 = xnode "Move a Fixed Distance"("Speed 1"=i8 50, "Distance 1"=90, "Motors"=w1242, "NXT/EV3"=w1243) -> ("NXT/EV3"=w1232:T3)
                            n297 = xnode "Motors"() -> ("Motor"=w1236:T2)
                            n298 = xnode "Move a Fixed Distance"("Speed 1"=i8 75, "Distance 1"=360, "Motors"=w1236, "NXT/EV3"=w1232) -> ("NXT/EV3"=w1233:T3)
                            n299 = xnode "Motors"() -> ("Motor"=w1239:T2)
                            n300 = xnode "Move a Fixed Distance"("Speed 1"=i8 75, "Distance 1"=-90, "Motors"=w1239, "NXT/EV3"=w1233) -> ()  [unwired: 1 out]
                          }
                        }
                      }
                      frame True {
                        n301 = local read "Large/Steel 2"() -> (w1292:dbl)
                        n302 = Decrement(x=w1292) -> (x-1=w1291:dbl)
                        n303 = local write "Large/Steel 2"(w1291) -> ()
                        n304 = xnode "Motors"() -> ("Motor"=w1293:T2)
                        n305 = xnode "Move a Fixed Distance"("Speed 1"=i8 75, "Distance 1"=360, "Motors"=w1293) -> ("NXT/EV3"=w1296:T3)  [unwired: 1 in]
                        n306 = xnode "Motors"() -> ("Motor"=w1297:T2)
                        n307 = xnode "Move a Fixed Distance"("Speed 1"=i8 50, "Distance 1"=90, "Motors"=w1297, "NXT/EV3"=w1296) -> ("NXT/EV3"=w1307:T3)
                        n308 = xnode "Motors"() -> ("Motor"=w1303:T2)
                        n309 = xnode "Move a Fixed Distance"("Speed 1"=i8 75, "Distance 1"=360, "Motors"=w1303, "NXT/EV3"=w1307) -> ("NXT/EV3"=w1306:T3)
                        n310 = xnode "Motors"() -> ("Motor"=w1300:T2)
                        n311 = xnode "Move a Fixed Distance"("Speed 1"=i8 75, "Distance 1"=-90, "Motors"=w1300, "NXT/EV3"=w1306) -> ()  [unwired: 1 out]
                      }
                    }
                  }
                  frame "Blue Glass" {
                    n312 = local read "Large/Steel 2"() -> (w1354:dbl)
                    n313 = Greater?(x=w1354, y=0.0) -> (0:w1353:bool)
                    n314 = case shown="False" w1353 {
                      frame True {
                        n315 = local read "Large/Steel 2"() -> (w1356:dbl)
                        n316 = Decrement(x=w1356) -> (x-1=w1355:dbl)
                        n317 = local write "Large/Steel 2"(w1355) -> ()
                        n318 = xnode "Motors"() -> ("Motor"=w1357:T2)
                        n319 = xnode "Move a Fixed Distance"("Speed 1"=i8 75, "Distance 1"=360, "Motors"=w1357) -> ("NXT/EV3"=w1360:T3)  [unwired: 1 in]
                        n320 = xnode "Motors"() -> ("Motor"=w1361:T2)
                        n321 = xnode "Move a Fixed Distance"("Speed 1"=i8 50, "Distance 1"=90, "Motors"=w1361, "NXT/EV3"=w1360) -> ("NXT/EV3"=w1371:T3)
                        n322 = xnode "Motors"() -> ("Motor"=w1367:T2)
                        n323 = xnode "Move a Fixed Distance"("Speed 1"=i8 75, "Distance 1"=360, "Motors"=w1367, "NXT/EV3"=w1371) -> ("NXT/EV3"=w1370:T3)
                        n324 = xnode "Motors"() -> ("Motor"=w1364:T2)
                        n325 = xnode "Move a Fixed Distance"("Speed 1"=i8 75, "Distance 1"=-90, "Motors"=w1364, "NXT/EV3"=w1370) -> ()  [unwired: 1 out]
                      }
                      frame False {
                        n326 = local read "Small/HDPE 2"() -> (w1418:dbl)
                        n327 = Greater?(x=w1418, y=0.0) -> (0:w1416:bool)
                        n328 = case shown="False" w1416 {
                          frame False {
                            (unwired) "This statement is false"
                          }
                          frame True {
                            n329 = local read "Small/HDPE 2"() -> (w1420:dbl)
                            n330 = Decrement(x=w1420) -> (x-1=w1419:dbl)
                            n331 = xnode "Motors"() -> ("Motor"=w1421:T2)
                            n332 = local write "Small/HDPE 2"(w1419) -> ()
                            n333 = xnode "Move a Fixed Distance"("Speed 1"=i8 75, "Distance 1"=360, "Motors"=w1421) -> ("NXT/EV3"=w1424:T3)  [unwired: 1 in]
                            n334 = xnode "Motors"() -> ("Motor"=w1425:T2)
                            n335 = xnode "Move a Fixed Distance"("Speed 1"=i8 50, "Distance 1"=90, "Motors"=w1425, "NXT/EV3"=w1424) -> ("NXT/EV3"=w1435:T3)
                            n336 = xnode "Motors"() -> ("Motor"=w1431:T2)
                            n337 = xnode "Move a Fixed Distance"("Speed 1"=i8 75, "Distance 1"=360, "Motors"=w1431, "NXT/EV3"=w1435) -> ("NXT/EV3"=w1434:T3)
                            n338 = xnode "Motors"() -> ("Motor"=w1428:T2)
                            n339 = xnode "Move a Fixed Distance"("Speed 1"=i8 75, "Distance 1"=-90, "Motors"=w1428, "NXT/EV3"=w1434) -> ()  [unwired: 1 out]
                          }
                        }
                      }
                    }
                  }
                  frame "Red Glass" {
                    n340 = local read "Large/Steel 2"() -> (w1482:dbl)
                    n341 = Greater?(x=w1482, y=0.0) -> (0:w1480:bool)
                    n342 = case shown="False" w1480 {
                      frame False {
                        n343 = local read "Small/HDPE 2"() -> (w1485:dbl)
                        n344 = Greater?(x=w1485, y=0.0) -> (0:w1483:bool)
                        n345 = case shown="False" w1483 {
                          frame False {
                            (unwired) "I hate everything\n"
                          }
                          frame True {
                            n346 = local read "Small/HDPE 2"() -> (w1487:dbl)
                            n347 = xnode "Motors"() -> ("Motor"=w1488:T2)
                            n348 = xnode "Move a Fixed Distance"("Speed 1"=i8 75, "Distance 1"=360, "Motors"=w1488) -> ("NXT/EV3"=w1491:T3)  [unwired: 1 in]
                            n349 = Decrement(x=w1487) -> (x-1=w1486:dbl)
                            n350 = local write "Small/HDPE 2"(w1486) -> ()
                            n351 = xnode "Motors"() -> ("Motor"=w1492:T2)
                            n352 = xnode "Move a Fixed Distance"("Speed 1"=i8 50, "Distance 1"=90, "Motors"=w1492, "NXT/EV3"=w1491) -> ("NXT/EV3"=w1502:T3)
                            n353 = xnode "Motors"() -> ("Motor"=w1498:T2)
                            n354 = xnode "Move a Fixed Distance"("Speed 1"=i8 75, "Distance 1"=360, "Motors"=w1498, "NXT/EV3"=w1502) -> ("NXT/EV3"=w1501:T3)
                            n355 = xnode "Motors"() -> ("Motor"=w1495:T2)
                            n356 = xnode "Move a Fixed Distance"("Speed 1"=i8 75, "Distance 1"=-90, "Motors"=w1495, "NXT/EV3"=w1501) -> ()  [unwired: 1 out]
                          }
                        }
                      }
                      frame True {
                        n357 = local read "Large/Steel 2"() -> (w1548:dbl)
                        n358 = Decrement(x=w1548) -> (x-1=w1547:dbl)
                        n359 = local write "Large/Steel 2"(w1547) -> ()
                        n360 = xnode "Motors"() -> ("Motor"=w1549:T2)
                        n361 = xnode "Move a Fixed Distance"("Speed 1"=i8 75, "Distance 1"=360, "Motors"=w1549) -> ("NXT/EV3"=w1552:T3)  [unwired: 1 in]
                        n362 = xnode "Motors"() -> ("Motor"=w1553:T2)
                        n363 = xnode "Move a Fixed Distance"("Speed 1"=i8 50, "Distance 1"=90, "Motors"=w1553, "NXT/EV3"=w1552) -> ("NXT/EV3"=w1563:T3)
                        n364 = xnode "Motors"() -> ("Motor"=w1559:T2)
                        n365 = xnode "Move a Fixed Distance"("Speed 1"=i8 75, "Distance 1"=360, "Motors"=w1559, "NXT/EV3"=w1563) -> ("NXT/EV3"=w1562:T3)
                        n366 = xnode "Motors"() -> ("Motor"=w1556:T2)
                        n367 = xnode "Move a Fixed Distance"("Speed 1"=i8 75, "Distance 1"=-90, "Motors"=w1556, "NXT/EV3"=w1562) -> ()  [unwired: 1 out]
                      }
                    }
                  }
                  frame "Steel/HDPE" {
                    n368 = local read "Large/Steel 2"() -> (w1610:dbl)
                    n369 = Greater?(x=w1610, y=0.0) -> (0:w1608:bool)
                    n370 = case shown="False" w1608 {
                      frame False {
                        n371 = local read "Small/HDPE 2"() -> (w1613:dbl)
                        n372 = Greater?(x=w1613, y=0.0) -> (0:w1611:bool)
                        n373 = case shown="False" w1611 {
                          frame False {
                            (unwired) "I've lost all my marbles"
                          }
                          frame True {
                            n374 = local read "Small/HDPE 2"() -> (w1615:dbl)
                            n375 = xnode "Motors"() -> ("Motor"=w1616:T2)
                            n376 = xnode "Move a Fixed Distance"("Speed 1"=i8 75, "Distance 1"=360, "Motors"=w1616) -> ("NXT/EV3"=w1619:T3)  [unwired: 1 in]
                            n377 = Decrement(x=w1615) -> (x-1=w1614:dbl)
                            n378 = local write "Small/HDPE 2"(w1614) -> ()
                            n379 = xnode "Motors"() -> ("Motor"=w1620:T2)
                            n380 = xnode "Move a Fixed Distance"("Speed 1"=i8 50, "Distance 1"=90, "Motors"=w1620, "NXT/EV3"=w1619) -> ("NXT/EV3"=w1630:T3)
                            n381 = xnode "Motors"() -> ("Motor"=w1626:T2)
                            n382 = xnode "Move a Fixed Distance"("Speed 1"=i8 75, "Distance 1"=360, "Motors"=w1626, "NXT/EV3"=w1630) -> ("NXT/EV3"=w1629:T3)
                            n383 = xnode "Motors"() -> ("Motor"=w1623:T2)
                            n384 = xnode "Move a Fixed Distance"("Speed 1"=i8 75, "Distance 1"=-90, "Motors"=w1623, "NXT/EV3"=w1629) -> ()  [unwired: 1 out]
                          }
                        }
                      }
                      frame True {
                        n385 = local read "Large/Steel 2"() -> (w1676:dbl)
                        n386 = Decrement(x=w1676) -> (x-1=w1675:dbl)
                        n387 = local write "Large/Steel 2"(w1675) -> ()
                        n388 = xnode "Motors"() -> ("Motor"=w1677:T2)
                        n389 = xnode "Move a Fixed Distance"("Speed 1"=i8 75, "Distance 1"=360, "Motors"=w1677) -> ("NXT/EV3"=w1680:T3)  [unwired: 1 in]
                        n390 = xnode "Motors"() -> ("Motor"=w1681:T2)
                        n391 = xnode "Move a Fixed Distance"("Speed 1"=i8 50, "Distance 1"=90, "Motors"=w1681, "NXT/EV3"=w1680) -> ("NXT/EV3"=w1691:T3)
                        n392 = xnode "Motors"() -> ("Motor"=w1687:T2)
                        n393 = xnode "Move a Fixed Distance"("Speed 1"=i8 75, "Distance 1"=360, "Motors"=w1687, "NXT/EV3"=w1691) -> ("NXT/EV3"=w1690:T3)
                        n394 = xnode "Motors"() -> ("Motor"=w1684:T2)
                        n395 = xnode "Move a Fixed Distance"("Speed 1"=i8 75, "Distance 1"=-90, "Motors"=w1684, "NXT/EV3"=w1690) -> ()  [unwired: 1 out]
                      }
                    }
                  }
                }
              }
            }
          }
          frame True {
            n396 = local read "Material 1"() -> (w1736:string)
            n397 = case shown="\"Blue Glass\"" w1736 {
              frame "White Glass", Default {
                n398 = local read "Large/Steel 1"() -> (w1738:dbl)
                n399 = Greater?(x=w1738, y=0.0) -> (0:w1737:bool)
                n400 = case shown="False" w1737 {
                  frame False {
                    n401 = local read "Small/HDPE 1"() -> (w1741:dbl)
                    n402 = Greater?(x=w1741, y=0.0) -> (0:w1740:bool)
                    n403 = case shown="True" w1740 {
                      frame False {
                        (unwired) "go away"
                      }
                      frame True {
                        n404 = xnode "Motors"() -> ("Motor"=w1743:T2)
                        n405 = xnode "Move a Fixed Distance"("Speed 1"=i8 75, "Distance 1"=360, "Motors"=w1743) -> ("NXT/EV3"=w1746:T3)  [unwired: 1 in]
                        n406 = local read "Small/HDPE 1"() -> (w1759:dbl)
                        n407 = Decrement(x=w1759) -> (x-1=w1758:dbl)
                        n408 = local write "Small/HDPE 1"(w1758) -> ()
                        n409 = xnode "Motors"() -> ("Motor"=w1747:T2)
                        n410 = xnode "Move a Fixed Distance"("Speed 1"=i8 50, "Distance 1"=90, "Motors"=w1747, "NXT/EV3"=w1746) -> ("NXT/EV3"=w1757:T3)
                        n411 = xnode "Motors"() -> ("Motor"=w1753:T2)
                        n412 = xnode "Move a Fixed Distance"("Speed 1"=i8 75, "Distance 1"=360, "Motors"=w1753, "NXT/EV3"=w1757) -> ("NXT/EV3"=w1756:T3)
                        n413 = xnode "Motors"() -> ("Motor"=w1750:T2)
                        n414 = xnode "Move a Fixed Distance"("Speed 1"=i8 75, "Distance 1"=-90, "Motors"=w1750, "NXT/EV3"=w1756) -> ()  [unwired: 1 out]
                      }
                    }
                  }
                  frame True {
                    n415 = local read "Large/Steel 1"() -> (w1820:dbl)
                    n416 = Decrement(x=w1820) -> (x-1=w1819:dbl)
                    n417 = xnode "Motors"() -> ("Motor"=w1804:T2)
                    n418 = xnode "Move a Fixed Distance"("Speed 1"=i8 75, "Distance 1"=360, "Motors"=w1804) -> ("NXT/EV3"=w1807:T3)  [unwired: 1 in]
                    n419 = local write "Large/Steel 1"(w1819) -> ()
                    n420 = xnode "Motors"() -> ("Motor"=w1808:T2)
                    n421 = xnode "Move a Fixed Distance"("Speed 1"=i8 50, "Distance 1"=90, "Motors"=w1808, "NXT/EV3"=w1807) -> ("NXT/EV3"=w1818:T3)
                    n422 = xnode "Motors"() -> ("Motor"=w1814:T2)
                    n423 = xnode "Move a Fixed Distance"("Speed 1"=i8 75, "Distance 1"=360, "Motors"=w1814, "NXT/EV3"=w1818) -> ("NXT/EV3"=w1817:T3)
                    n424 = xnode "Motors"() -> ("Motor"=w1811:T2)
                    n425 = xnode "Move a Fixed Distance"("Speed 1"=i8 75, "Distance 1"=-90, "Motors"=w1811, "NXT/EV3"=w1817) -> ()  [unwired: 1 out]
                  }
                }
              }
              frame "Red Glass" {
                n426 = local read "Large/Steel 1"() -> (w1867:dbl)
                n427 = Greater?(x=w1867, y=0.0) -> (0:w1866:bool)
                n428 = case shown="False" w1866 {
                  frame False {
                    n429 = local read "Small/HDPE 1"() -> (w1870:dbl)
                    n430 = Greater?(x=w1870, y=0.0) -> (0:w1868:bool)
                    n431 = case shown="True" w1868 {
                      frame False {
                        (unwired) "donezo"
                      }
                      frame True {
                        n432 = xnode "Motors"() -> ("Motor"=w1871:T2)
                        n433 = local read "Small/HDPE 1"() -> (w1887:dbl)
                        n434 = xnode "Move a Fixed Distance"("Speed 1"=i8 75, "Distance 1"=360, "Motors"=w1871) -> ("NXT/EV3"=w1874:T3)  [unwired: 1 in]
                        n435 = Decrement(x=w1887) -> (x-1=w1886:dbl)
                        n436 = local write "Small/HDPE 1"(w1886) -> ()
                        n437 = xnode "Motors"() -> ("Motor"=w1875:T2)
                        n438 = xnode "Move a Fixed Distance"("Speed 1"=i8 50, "Distance 1"=90, "Motors"=w1875, "NXT/EV3"=w1874) -> ("NXT/EV3"=w1885:T3)
                        n439 = xnode "Motors"() -> ("Motor"=w1881:T2)
                        n440 = xnode "Move a Fixed Distance"("Speed 1"=i8 75, "Distance 1"=360, "Motors"=w1881, "NXT/EV3"=w1885) -> ("NXT/EV3"=w1884:T3)
                        n441 = xnode "Motors"() -> ("Motor"=w1878:T2)
                        n442 = xnode "Move a Fixed Distance"("Speed 1"=i8 75, "Distance 1"=-90, "Motors"=w1878, "NXT/EV3"=w1884) -> ()  [unwired: 1 out]
                      }
                    }
                  }
                  frame True {
                    n443 = local read "Large/Steel 1"() -> (w1948:dbl)
                    n444 = Decrement(x=w1948) -> (x-1=w1947:dbl)
                    n445 = xnode "Motors"() -> ("Motor"=w1932:T2)
                    n446 = xnode "Move a Fixed Distance"("Speed 1"=i8 75, "Distance 1"=360, "Motors"=w1932) -> ("NXT/EV3"=w1935:T3)  [unwired: 1 in]
                    n447 = local write "Large/Steel 1"(w1947) -> ()
                    n448 = xnode "Motors"() -> ("Motor"=w1936:T2)
                    n449 = xnode "Move a Fixed Distance"("Speed 1"=i8 50, "Distance 1"=90, "Motors"=w1936, "NXT/EV3"=w1935) -> ("NXT/EV3"=w1946:T3)
                    n450 = xnode "Motors"() -> ("Motor"=w1942:T2)
                    n451 = xnode "Move a Fixed Distance"("Speed 1"=i8 75, "Distance 1"=360, "Motors"=w1942, "NXT/EV3"=w1946) -> ("NXT/EV3"=w1945:T3)
                    n452 = xnode "Motors"() -> ("Motor"=w1939:T2)
                    n453 = xnode "Move a Fixed Distance"("Speed 1"=i8 75, "Distance 1"=-90, "Motors"=w1939, "NXT/EV3"=w1945) -> ()  [unwired: 1 out]
                  }
                }
              }
              frame "Blue Glass" {
                n454 = local read "Large/Steel 1"() -> (w1995:dbl)
                n455 = Greater?(x=w1995, y=0.0) -> (0:w1993:bool)
                n456 = case shown="False" w1993 {
                  frame False {
                    n457 = local read "Small/HDPE 1"() -> (w1997:dbl)
                    n458 = Greater?(x=w1997, y=0.0) -> (0:w1998:bool)
                    n459 = case shown="True" w1998 {
                      frame False {
                        (unwired) "Welcome to labview hell"
                      }
                      frame True {
                        n460 = local read "Small/HDPE 1"() -> (w2015:dbl)
                        n461 = xnode "Motors"() -> ("Motor"=w1999:T2)
                        n462 = xnode "Move a Fixed Distance"("Speed 1"=i8 75, "Distance 1"=360, "Motors"=w1999) -> ("NXT/EV3"=w2002:T3)  [unwired: 1 in]
                        n463 = Decrement(x=w2015) -> (x-1=w2014:dbl)
                        n464 = xnode "Motors"() -> ("Motor"=w2003:T2)
                        n465 = xnode "Move a Fixed Distance"("Speed 1"=i8 50, "Distance 1"=90, "Motors"=w2003, "NXT/EV3"=w2002) -> ("NXT/EV3"=w2013:T3)
                        n466 = local write "Small/HDPE 1"(w2014) -> ()
                        n467 = xnode "Motors"() -> ("Motor"=w2009:T2)
                        n468 = xnode "Move a Fixed Distance"("Speed 1"=i8 75, "Distance 1"=360, "Motors"=w2009, "NXT/EV3"=w2013) -> ("NXT/EV3"=w2012:T3)
                        n469 = xnode "Motors"() -> ("Motor"=w2006:T2)
                        n470 = xnode "Move a Fixed Distance"("Speed 1"=i8 75, "Distance 1"=-90, "Motors"=w2006, "NXT/EV3"=w2012) -> ()  [unwired: 1 out]
                      }
                    }
                  }
                  frame True {
                    n471 = xnode "Motors"() -> ("Motor"=w2062:T2)
                    n472 = local read "Large/Steel 1"() -> (w2061:dbl)
                    n473 = xnode "Move a Fixed Distance"("Speed 1"=i8 75, "Distance 1"=360, "Motors"=w2062) -> ("NXT/EV3"=w2065:T3)  [unwired: 1 in]
                    n474 = Decrement(x=w2061) -> (x-1=w2060:dbl)
                    n475 = xnode "Motors"() -> ("Motor"=w2066:T2)
                    n476 = xnode "Move a Fixed Distance"("Speed 1"=i8 50, "Distance 1"=90, "Motors"=w2066, "NXT/EV3"=w2065) -> ("NXT/EV3"=w2076:T3)
                    n477 = local write "Large/Steel 1"(w2060) -> ()
                    n478 = xnode "Motors"() -> ("Motor"=w2072:T2)
                    n479 = xnode "Move a Fixed Distance"("Speed 1"=i8 75, "Distance 1"=360, "Motors"=w2072, "NXT/EV3"=w2076) -> ("NXT/EV3"=w2075:T3)
                    n480 = xnode "Motors"() -> ("Motor"=w2069:T2)
                    n481 = xnode "Move a Fixed Distance"("Speed 1"=i8 75, "Distance 1"=-90, "Motors"=w2069, "NXT/EV3"=w2075) -> ()  [unwired: 1 out]
                  }
                }
              }
              frame "Steel/HDPE" {
                n482 = local read "Large/Steel 1"() -> (w2123:dbl)
                n483 = Greater?(x=w2123, y=0.0) -> (0:w2122:bool)
                n484 = case shown="False" w2122 {
                  frame False {
                    n485 = local read "Small/HDPE 1"() -> (w2126:dbl)
                    n486 = Greater?(x=w2126, y=0.0) -> (0:w2125:bool)
                    n487 = case shown="True" w2125 {
                      frame False {
                        (unwired) "why are you even here"
                      }
                      frame True {
                        n488 = local read "Small/HDPE 1"() -> (w2128:dbl)
                        n489 = xnode "Motors"() -> ("Motor"=w2129:T2)
                        n490 = Decrement(x=w2128) -> (x-1=w2127:dbl)
                        n491 = xnode "Move a Fixed Distance"("Speed 1"=i8 75, "Distance 1"=360, "Motors"=w2129) -> ("NXT/EV3"=w2132:T3)  [unwired: 1 in]
                        n492 = local write "Small/HDPE 1"(w2127) -> ()
                        n493 = xnode "Motors"() -> ("Motor"=w2133:T2)
                        n494 = xnode "Move a Fixed Distance"("Speed 1"=i8 50, "Distance 1"=90, "Motors"=w2133, "NXT/EV3"=w2132) -> ("NXT/EV3"=w2143:T3)
                        n495 = xnode "Motors"() -> ("Motor"=w2139:T2)
                        n496 = xnode "Move a Fixed Distance"("Speed 1"=i8 75, "Distance 1"=360, "Motors"=w2139, "NXT/EV3"=w2143) -> ("NXT/EV3"=w2142:T3)
                        n497 = xnode "Motors"() -> ("Motor"=w2136:T2)
                        n498 = xnode "Move a Fixed Distance"("Speed 1"=i8 75, "Distance 1"=-90, "Motors"=w2136, "NXT/EV3"=w2142) -> ()  [unwired: 1 out]
                      }
                    }
                  }
                  frame True {
                    n499 = local read "Large/Steel 1"() -> (w2189:dbl)
                    n500 = Decrement(x=w2189) -> (x-1=w2188:dbl)
                    n501 = xnode "Motors"() -> ("Motor"=w2204:T2)
                    n502 = xnode "Move a Fixed Distance"("Speed 1"=i8 75, "Distance 1"=360, "Motors"=w2204) -> ("NXT/EV3"=w2201:T3)  [unwired: 1 in]
                    n503 = local write "Large/Steel 1"(w2188) -> ()
                    n504 = xnode "Motors"() -> ("Motor"=w2200:T2)
                    n505 = xnode "Move a Fixed Distance"("Speed 1"=i8 50, "Distance 1"=90, "Motors"=w2200, "NXT/EV3"=w2201) -> ("NXT/EV3"=w2190:T3)
                    n506 = xnode "Motors"() -> ("Motor"=w2194:T2)
                    n507 = xnode "Move a Fixed Distance"("Speed 1"=i8 75, "Distance 1"=360, "Motors"=w2194, "NXT/EV3"=w2190) -> ("NXT/EV3"=w2191:T3)
                    n508 = xnode "Motors"() -> ("Motor"=w2197:T2)
                    n509 = xnode "Move a Fixed Distance"("Speed 1"=i8 75, "Distance 1"=-90, "Motors"=w2197, "NXT/EV3"=w2191) -> ()  [unwired: 1 out]
                  }
                }
              }
            }
          }
        }
      }
    }
  }
